vi "采配水模拟器.vi"() -> ()   [LabVIEW 2016, in "采配水.lvlib"]
uses:
  <vilib>/NI/Modbus Library/Network Protocol/Network Slave/daemon status.ctl
  <vilib>/NI/Modbus Library/Network Protocol/Network Slave/TCP/Connection.ctl
  <vilib>/Plasmionique/MB Master/MB_Master_TCP/MB_Master_TCP.lvclass
  C:/Program Files (x86)/National Instruments/LabVIEW 2016/vi.lib/Plasmionique/MB Master/MB_Master/MB_Master.lvclass
  <vilib>/NI/Modbus Library/API/Wrapper/Create TCP Slave.vi
  <vilib>/NI/Modbus Library/API/slave/Modbus Slave.lvclass
  <vilib>/NI/Modbus Library/API/Wrapper/API Main.lvlib
  <vilib>/NI/Modbus Library/Network Protocol/Network Slave/Network Slave.lvclass
  <vilib>/NI/Modbus Library/Network Protocol/Network Slave/TCP/TCP Slave.lvclass
panel:
  out "Session Valid":bool
  out "TCP Connection List":T1[](array[typedef])
  out "TCP Connection Count":u32
  out "Daemon Status":T2
  out "Daemon Error":errorcluster
  out "启动/停止命令":enum16{"待机", "水样测试", "停止", "加标回收"}(ring)
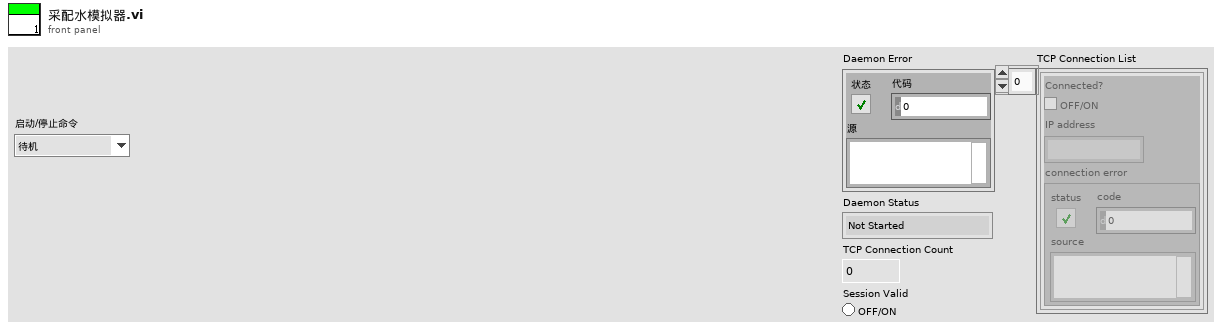
[diagram p1: front panel]
types:
  T1 = typedef "TCP Slave.lvclass/Connection.ctl" = cluster{"Connected?":bool, "IP address":string, "connection error":errorcluster}
  T2 = typedef "Network Slave.lvclass/daemon status.ctl" = enum16{"Not Started", "Running", "Error", "Stopped"}
  T3 = typedef "采配水.lvlib/采配水流程.ctl" = u16
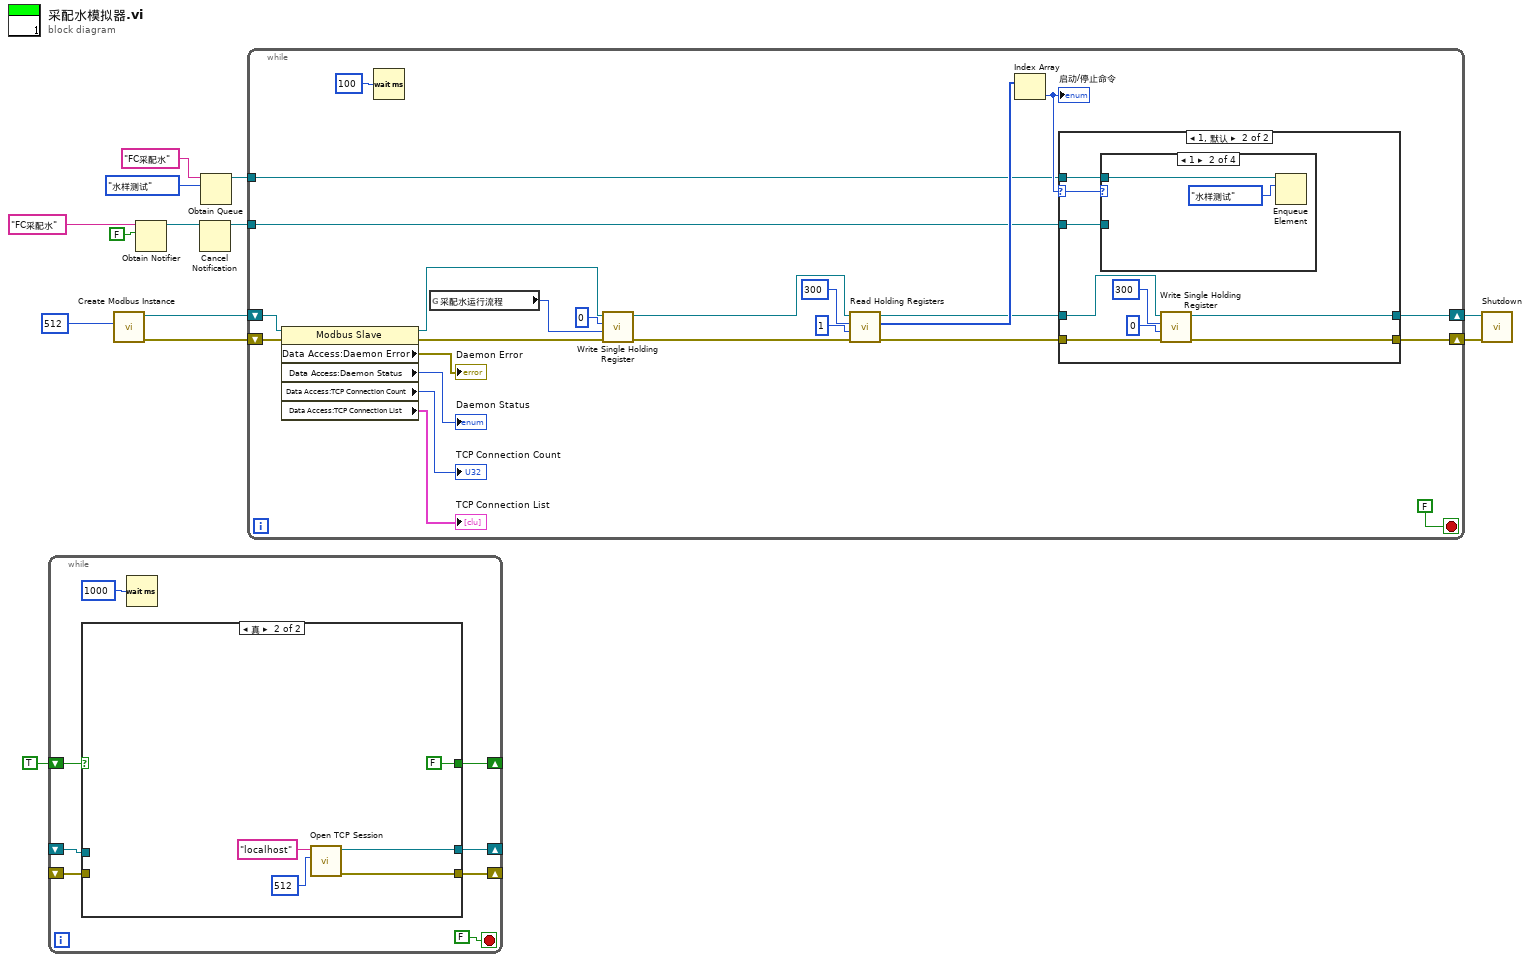
[diagram p0: block diagram]
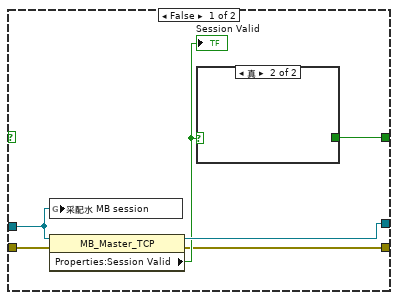
[diagram p2: hidden frame]
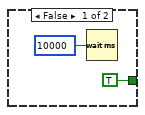
[diagram p3: hidden frame]
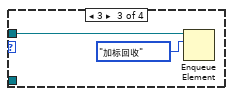
[diagram p6: hidden frame]
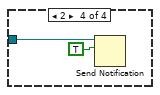
[diagram p7: hidden frame]
diagram:
  n1 = while {
    shift-right: [w21] -> _
    shift-left: _ -> [w20]
    shift-right: [w15] -> _
    shift-left: TRUE -> [w17]
    shift-right: [w18] -> _
    shift-left: _ -> [w16]
    stop <- FALSE stop-if-true
    n2 = case shown="真" w17 {
      tunnel: [w27 w34] -> w21
      tunnel: w20 -> [w22 _]
      tunnel: [w23 w31] -> w18
      tunnel: w16 -> [w24 _]
      tunnel: [w25 FALSE] -> w15
      frame False {
        n3 = global write "通讯全局变量.vi" "采配水 MB session"(w22) -> ()
        n4 = property class="MB_Master_TCP"(reference=w22, error in=w24) -> (reference out=w27:refnum<class "MB_Master_TCP.lvclass">, error out=w23:errorcluster, "Properties:Session Valid"=w26:bool)
        "Session Valid" <- w26
        n5 = case shown="真" w26 {
          tunnel: [TRUE _] -> w25
          frame False {
            n6 = Wait (ms)(milliseconds to wait=u32 10000 ("等待时间（毫秒）")) -> ()  [unwired: 1 out]
          }
          frame True {
          }
        }
      }
      frame True {
        n7 = call <vilib>:"Open TCP Session.vi"("Port (502)"=u16 512, "IP Address"="localhost") -> ("error out"=w31:errorcluster, "MB_TCP session"=w34:refnum<class "MB_Master_TCP.lvclass">)  [unwired: 8 in]
      }
    }
    n8 = Wait (ms)(milliseconds to wait=u32 1000 ("等待时间（毫秒）")) -> ()  [unwired: 1 out]
  }
  n9 = call-poly <vilib>:"Create Modbus Instance.vi"("port (502)"=u16 512) -> ("error out"=w11:errorcluster, "TCP slave instance"=w13:refnum<class "Modbus Slave.lvclass">)  [unwired: 9 in]
  n10 = Obtain Notifier(name (unnamed)="FC采配水" ("名称（未命名）"), notification data type=FALSE) -> (notifier out=w3:refnum<notifier>)  [unwired: 2 in, 2 out]
  n11 = Cancel Notification(0:w3) -> (8:w2:refnum<notifier>)  [unwired: 1 in, 2 out]
  n12 = Obtain Queue(name (unnamed)="FC采配水" ("名称（未命名）"), element data type=enum16{"水样测试", "加标回收"}."水样测试" ("启动类型")) -> (queue out=w6:refnum<queue>)  [unwired: 3 in, 2 out]
  n13 = while {
    shift-right: [w51] -> w12
    shift-left: w13 -> [w45]
    shift-right: [w46] -> w10
    shift-left: w11 -> [w44]
    tunnel: w6 -> [w36]
    tunnel: w2 -> [w35]
    stop <- FALSE stop-if-true
    n14 = property class="Modbus Slave"(reference=w45, error in=w44) -> (reference out=w42:refnum<class "Modbus Slave.lvclass">, error out=w43:errorcluster, "Data Access:Daemon Error"=→"Daemon Error":errorcluster, "Data Access:Daemon Status"=→"Daemon Status":T2, "Data Access:TCP Connection Count"=→"TCP Connection Count":u32, "Data Access:TCP Connection List"=→"TCP Connection List":T1[])
    n15 = Wait (ms)(milliseconds to wait=u32 100 ("等待时间（毫秒）")) -> ()  [unwired: 1 out]
    n16 = global read "通讯全局变量.vi" "采配水运行流程"() -> (w37:T3)
    n17 = call-dynamic "Write Single Holding Register.vi"("error in"=w43, "register to write"=w37, "address"=u16 0, "Modbus slave in"=w42) -> ("error out"=w48:errorcluster, "Modbus slave out"=w49:refnum<class "Modbus Slave.lvclass">)  [unwired: 6 in]
    n18 = call-dynamic "Read Holding Registers.vi"("error in"=w48, "number of inputs"=u16 1, "starting address"=u16 300, "Modbus slave in"=w49) -> ("error out"=w50:errorcluster, "register values"=w54:u16[], "Modbus slave out"=w52:refnum<class "Modbus Slave.lvclass">)  [unwired: 5 in]
    n19 = Index Array(array=w54) -> (element=w53:u16)  [unwired: 1 in]
    "启动/停止命令" <- w53
    n20 = case shown="1, 默认" w53 {
      selector: w53 -> [_ w63]
      tunnel: w52 -> [w60 w69]
      tunnel: [w60 w68] -> w51
      tunnel: w50 -> [w59 w67]
      tunnel: [w59 w66] -> w46
      tunnel: w36 -> [_ w62]
      tunnel: w35 -> [_ w61]
      frame 0 {
      }
      frame 1, Default {
        n21 = case shown="1" w63 {
          tunnel: w62 -> [_ w71 w73 _]
          tunnel: w61 -> [_ _ _ w75]
          frame 0, Default {
          }
          frame 1 {
            n22 = Enqueue Element(queue=w71, element=enum16{"水样测试", "加标回收"}."水样测试" ("元素")) -> ()  [unwired: 2 in, 3 out]
          }
          frame 3 {
            n23 = Enqueue Element(queue=w73, element=enum16{"水样测试", "加标回收"}."加标回收" ("元素")) -> ()  [unwired: 2 in, 3 out]
          }
          frame 2 {
            n24 = Send Notification(notification=TRUE ("通知"), notifier=w75) -> ()  [unwired: 1 in, 2 out]
          }
        }
        n25 = call-dynamic "Write Single Holding Register.vi"("error in"=w67, "register to write"=u16 0, "address"=u16 300, "Modbus slave in"=w69) -> ("error out"=w66:errorcluster, "Modbus slave out"=w68:refnum<class "Modbus Slave.lvclass">)  [unwired: 6 in]
      }
    }
  }
  n26 = call-dynamic "Shutdown.vi"("error in"=w10, "Modbus slave in"=w12) -> ()  [unwired: 9 in, 1 out]
